vi "rs3_CropRGB_BW.vi"(0 "RGB Array":u8[](array[numeric])=array[1221120 elements], 1 "start Y":i32, 3 "Output Height Y":i32, 5 "Color format":enum16{"Monochrome", "RGB internal (RGB)"}(ring), 7 "Input Height Y":i32=480, 9 "Input Width X":i32=848, 11 "Zoom":bool=TRUE, 12 "Start X":i32, 14 "Output Width X":i32) -> (4 "New RGB Array":u8[](array[numeric]))   [LabVIEW 2017, in "libRealSense3.lvlib"]
uses:
  libRealSense3.lvlib
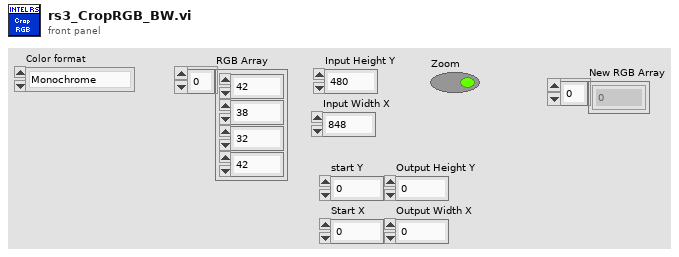
[diagram p1: front panel]
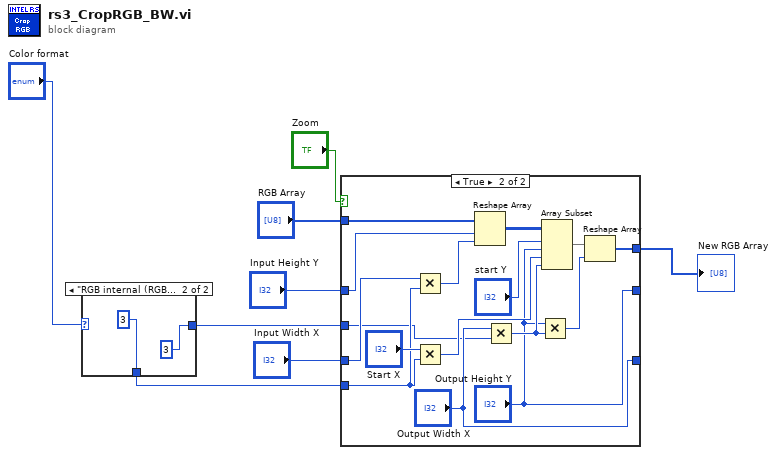
[diagram p0: block diagram]
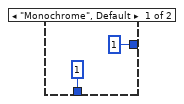
[diagram p2: hidden frame]
diagram:
  n1 = case shown="\"RGB internal (RGB)\"" "Color format" {
    tunnel: [1 ("y") 3 ("y")] -> w3
    tunnel: [1 ("y") 3 ("y")] -> w2
    frame "Monochrome", Default {
    }
    frame "RGB internal (RGB)" {
    }
  }
  n2 = case shown="True" "Zoom" {
    tunnel: "RGB Array" -> [w15 w28]
    tunnel: "Input Height Y" -> [w14 w27]
    tunnel: [w15 w25] -> w6
    tunnel: "Input Width X" -> [w13 w24]
    tunnel: [w14 "Output Height Y"] -> _
    tunnel: [w13 "Output Width X"] -> _
    tunnel: w3 -> [_ w17]
    tunnel: w2 -> [_ w16]
    frame False {
    }
    frame True {
      n3 = Multiply(x=w24, y=w17) -> (x*y=w23:i32)
      n4 = Multiply(x="Start X", y=w17) -> (x*y=w21:i32)
      n5 = Reshape Array(w28, w27, w23) -> (w26:u8[][])
      n6 = Multiply(x="Output Width X", y=w16) -> (x*y=w20:i32)
      n7 = Multiply(x="Output Height Y", y=w20) -> (x*y=w29:i32)
      n8 = Array Subset(array=w26, index (row)="start Y", length (row)="Output Height Y", index (col)=w21, length (col)=w20) -> (w30:u8[][])
      n9 = Reshape Array(w30, w29) -> (w25:u8[])
    }
  }
  "New RGB Array" <- w6
